vi "Test Breakpoints Roundtrip.vi"() -> (0 "error out":errorcluster)   [LabVIEW 2020]
doc: "Test setting and retreiving of breakpoints."
uses:
  <vilib>/addons/_JKI Toolkits/Caraya/classes/Test/Test.lvclass
  <vilib>/addons/_JKI Toolkits/Caraya/classes/Assert/Assert.lvclass
  src/Type Definitions/Class Name--enum.ctl
  <vilib>/Utility/miscctls.llb/LVBreakpointStatusEnum.ctl
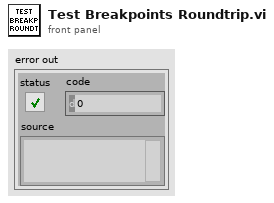
[diagram p1: front panel]
types:
  T1 = typedef "Class Name--enum.ctl" = enum16{"Node", "Wire"}
  T2 = typedef "Breakpoint--cluster.ctl" = cluster{"UID":i32, "BP Status":T3, "Class Name":T1}
  T3 = typedef "LVBreakpointStatusEnum.ctl" = enum8{"Cleared Break", "Enabled Break", "Disabled Break"}
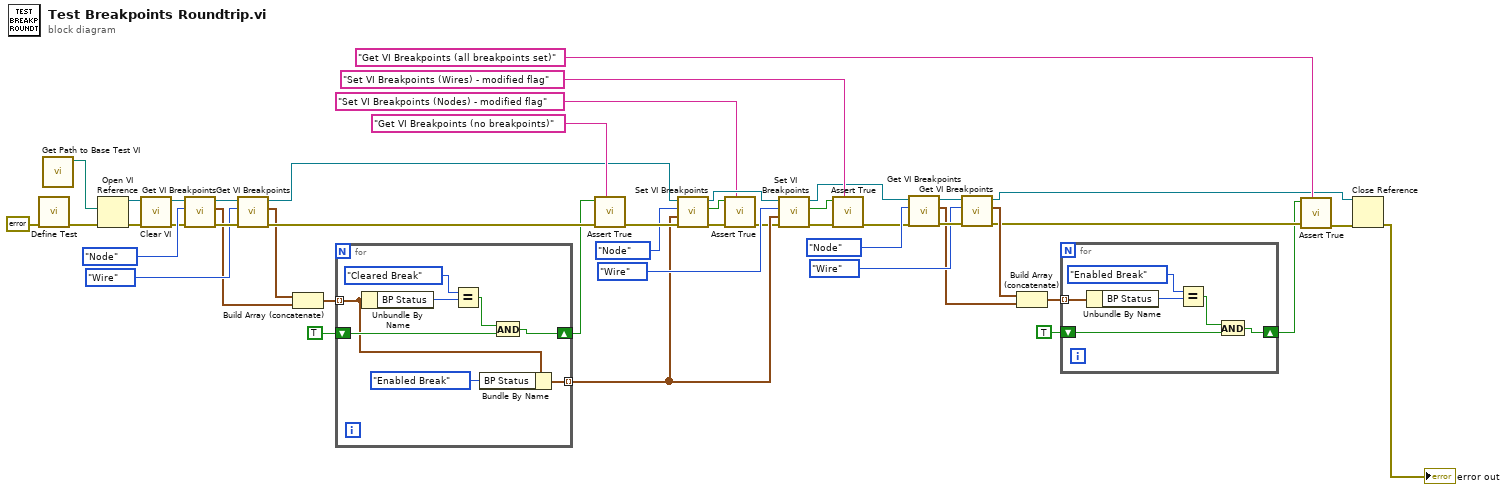
[diagram p0: block diagram]
diagram:
  n1 = call <vilib>:"Define Test.vi"("error in (no error)"=errorcluster {"status"=FALSE, "code"=0, "source"=""}) -> ("error out"=w4:errorcluster)  [unwired: 9 in, 1 out]
  n2 = call "Get Path to Base Test VI.vi"() -> ("Path"=w45:path)  [unwired: 11 in]
  n3 = Open VI Reference(vi path=w45, error in (no error)=w4) -> (vi reference=w2:refnum<vi>, error out=w44:errorcluster)  [unwired: 4 in]
  n4 = call "Clear VI.vi"("error in"=w44, "VI Refnum In"=w2) -> ("error out"=w3:errorcluster, "VI Refnum Out"=w1:refnum<vi>)  [unwired: 8 in]
  n5 = call "Get VI Breakpoints.vi"("error in"=w3, "Class Name"=Class_Name--enum."Node", "VI Reference in"=w1) -> ("error out"=w42:errorcluster, "Breakpoints"=w36:T2[], "VI Reference out"=w39:refnum<vi>)  [unwired: 6 in]
  n6 = call "Get VI Breakpoints.vi"("error in"=w42, "Class Name"=Class_Name--enum."Wire", "VI Reference in"=w39) -> ("error out"=w40:errorcluster, "Breakpoints"=w37:T2[], "VI Reference out"=w31:refnum<vi>)  [unwired: 6 in]
  n7 = Build Array (concatenate)(w37, w36) -> (w35:T2[])
  n8 = for {
    tunnel: w35 -> [w50] mode=indexing
    shift-right: [w51] -> w33
    shift-left: TRUE -> [w55]
    tunnel: [w48] -> w27 mode=indexing
    n9 = Unbundle By Name(w50) -> ("BP Status"=w53:T3)
    n10 = Equal?(x=LVBreakpointStatusEnum."Cleared Break", y=w53) -> (x = y?=w54:bool)
    n11 = Bundle By Name(cluster=w50, "BP Status"=LVBreakpointStatusEnum."Enabled Break") -> (w48:T2)
    n12 = And(x=w54, y=w55) -> (x .and. y?=w51:bool)
  }
  n13 = call <vilib>:"Assert True.vi"("Label"="Get VI Breakpoints (no breakpoints)", "error in (no error)"=w40, "True?"=w33) -> ("error out"=w32:errorcluster)  [unwired: 7 in, 1 out]
  n14 = call "Set VI Breakpoints.vi"("error in"=w32, "Breakpoints"=w27, "Class Name"=Class_Name--enum."Node", "VI Reference in"=w31) -> ("error out"=w26:errorcluster, "VI Modified"=w5:bool, "VI Reference out"=w29:refnum<vi>)  [unwired: 5 in]
  n15 = call <vilib>:"Assert True.vi"("Label"="Set VI Breakpoints (Nodes) - modified flag", "error in (no error)"=w26, "True?"=w5) -> ("error out"=w25:errorcluster)  [unwired: 7 in, 1 out]
  n16 = call "Set VI Breakpoints.vi"("error in"=w25, "Breakpoints"=w27, "Class Name"=Class_Name--enum."Wire", "VI Reference in"=w29) -> ("error out"=w23:errorcluster, "VI Modified"=w22:bool, "VI Reference out"=w16:refnum<vi>)  [unwired: 5 in]
  n17 = call <vilib>:"Assert True.vi"("Label"="Set VI Breakpoints (Wires) - modified flag", "error in (no error)"=w23, "True?"=w22) -> ("error out"=w15:errorcluster)  [unwired: 7 in, 1 out]
  n18 = call "Get VI Breakpoints.vi"("error in"=w15, "Class Name"=Class_Name--enum."Node", "VI Reference in"=w16) -> ("error out"=w20:errorcluster, "Breakpoints"=w12:T2[], "VI Reference out"=w18:refnum<vi>)  [unwired: 6 in]
  n19 = call "Get VI Breakpoints.vi"("error in"=w20, "Class Name"=Class_Name--enum."Wire", "VI Reference in"=w18) -> ("error out"=w11:errorcluster, "Breakpoints"=w17:T2[], "VI Reference out"=w6:refnum<vi>)  [unwired: 6 in]
  n20 = Build Array (concatenate)(w17, w12) -> (w13:T2[])
  n21 = for {
    tunnel: w13 -> [w56] mode=indexing
    shift-right: [w57] -> w10
    shift-left: TRUE -> [w61]
    n22 = Unbundle By Name(w56) -> ("BP Status"=w59:T3)
    n23 = Equal?(x=LVBreakpointStatusEnum."Enabled Break", y=w59) -> (x = y?=w60:bool)
    n24 = And(x=w60, y=w61) -> (x .and. y?=w57:bool)
  }
  n25 = call <vilib>:"Assert True.vi"("Label"="Get VI Breakpoints (all breakpoints set)", "error in (no error)"=w11, "True?"=w10) -> ("error out"=w7:errorcluster)  [unwired: 7 in, 1 out]
  n26 = Close Reference(reference=w6, error in (no error)=w7) -> (error out=→"error out":errorcluster)
